vi "Heartbeat stop.vi"(4 "error in":errorcluster, 6 "Node ID":u8, 7 "CANopen in":refnum<class "CANopen.lvclass">) -> (0 "error out":errorcluster, 3 "CANopen out":refnum<class "CANopen.lvclass">)   [LabVIEW 2026, in "canopen_.lvlib" / "CANopen.lvclass"]
doc: "Stops the generation of heartbeat messages on a specific CANopen node or on all nodes in the heartbeat table if \"Node ID\" is not specified."
uses:
  CANopen.lvclass
  CANopen.lvclass/CANopen.ctl
  Multiplexor.ctl
  CANopen Master.lvlib
  SDO download (U16).vi
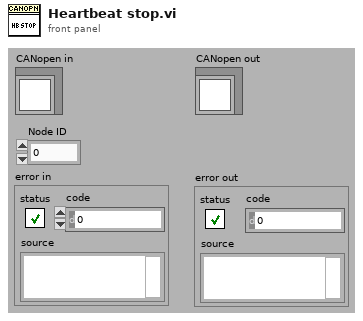
[diagram p1: front panel]
types:
  T1 = cluster{"Node ID":u8, "Period":u16, "Timeout":u16, "Last Beat":timestamp}[]
  T2 = typedef "CANopen Master.lvlib/Multiplexor.ctl" = cluster{"Index":u16, "Sub-Index":i16}
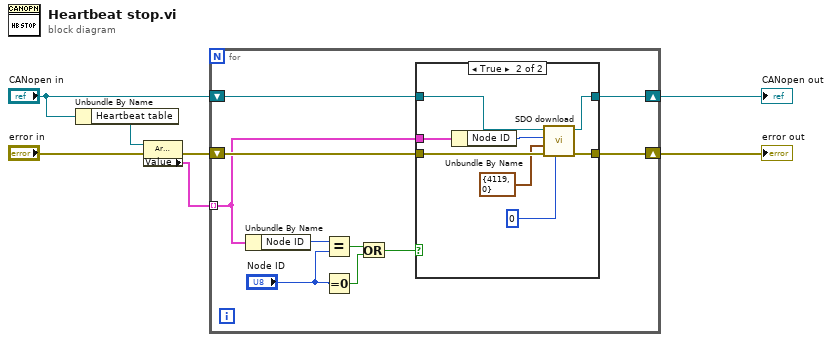
[diagram p0: block diagram]
diagram:
  n1 = Unbundle By Name("CANopen in") -> ("Heartbeat table"=w7:refnum<vi>)
  n2 = property class="Arr (strict)"(reference=w7, error in="error in") -> (error out=w3:errorcluster, "Value"=w6:T1)  [unwired: 1 out]
  n3 = for {
    tunnel: w6 -> [w10] mode=indexing
    shift-right: [w13] -> w2
    shift-left: w3 -> [w14]
    shift-right: [w8] -> w1
    shift-left: "CANopen in" -> [w12]
    n4 = Unbundle By Name(w10) -> ("Node ID"=w11:u8)
    n5 = Equal?(x=w11, y="Node ID") -> (x = y?=w16:bool)
    n6 = Equal To 0?(x="Node ID") -> (x = 0?=w15:bool)
    n7 = Or(x=w16, y=w15) -> (x .or. y?=w9:bool)
    n8 = case shown="True" w9 {
      tunnel: w14 -> [w19 w27]
      tunnel: [w19 w26] -> w13
      tunnel: w12 -> [w18 w22]
      tunnel: w10 -> [_ w24]
      tunnel: [w18 w21] -> w8
      frame False {
      }
      frame True {
        n9 = Unbundle By Name(w24) -> ("Node ID"=w23:u8)
        n10 = call-poly "SDO download.vi"("Value"=i16 0, "error in (no error)"=w27, "Multiplexor"=T2 {"Index"=4119, "Sub-Index"=0}, "Node ID"=w23, "CANopen in"=w22) -> ("error out"=w26:errorcluster, "CANopen out"=w21:refnum<class "CANopen.lvclass">)  [unwired: 1 in, 2 out]
      }
    }
  }
  "CANopen out" <- w1
  "error out" <- w2
